vi "MCS_Go to Marked Zero.vi"() -> ()   [LabVIEW 2010]
panel:
  out "error out":errorcluster
  in  "error in (no error)":errorcluster
  in  "MCS System Locator":string
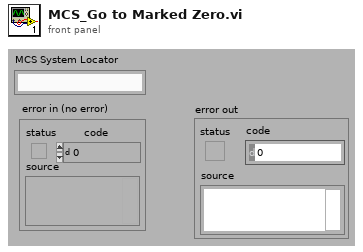
[diagram p1: front panel]
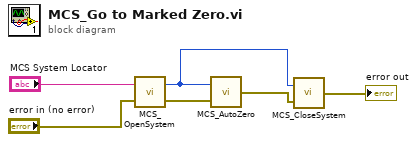
[diagram p0: block diagram]
diagram:
  n1 = call "MCS_OpenSystem.vi"("error in (no error)"="error in (no error)", "MCS System Locator"="MCS System Locator") -> ("error out"=w4:errorcluster, "System Index Out"=w3:u32)
  n2 = call "MCS_AutoZero.vi"("error in (no error)"=w4, "System Index In"=w3) -> ("error out"=w2:errorcluster)
  n3 = call "MCS_CloseSystem.vi"("error in (no error)"=w2, "System Index In"=w3) -> ("error out"=→"error out":errorcluster)
